vi "LV SCISDK Free Lib.vi"(8 "error in (no error)":errorcluster, 11 "handle":u64) -> (0 "error out":errorcluster, 3 "function return":i32)   [LabVIEW 2021, in "SciSDK_Labview.lvlib"]
doc: "You need this VI to free up library instance's memory"
uses:
  SciSDK_Labview.lvlib
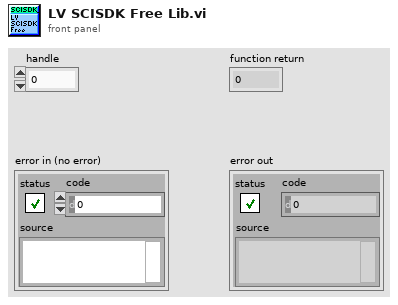
[diagram p1: front panel]
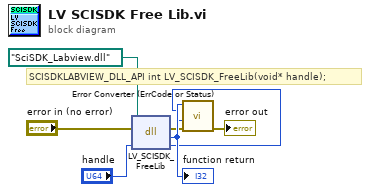
[diagram p0: block diagram]
diagram:
  # "SCISDKLABVIEW_DLL_API int LV_SCISDK_FreeLib(void* handle);"
  n1 = dll-call lib="C:/git/scisdk/SciSDK_VC++/x64/Debug/SciSDK_Labview.*" fn="LV_SCISDK_FreeLib"(path in=path "SciSDK_Labview.dll", error in="error in (no error)", "handle"="handle") -> (error out=w4:errorcluster, "return type"=w7:i32, "handle"=w1:u64)  [unwired: 1 in, 1 out]
  "function return" <- w7
  n2 = call "Error Converter (ErrCode or Status).vi"("error in (no error)"=w4, "handle"=w1, "error code"=w7) -> ("error out"=→"error out":errorcluster)  [unwired: 8 in]
